vi "Stop Server.vi"(8 "error in (no error)":errorcluster, 11 "OOP Server in":refnum<class "Template Server.lvclass">) -> (0 "error out":errorcluster, 3 "OOP Server out":refnum<class "Template Server.lvclass">)   [LabVIEW 2019, in "Template Server.lvlib" / "Template Server.lvclass"]
uses:
  Template Server.lvclass
  Template Server.lvclass/Template Server.ctl
  gRPC interface/gprc-lvsupport.lvlib
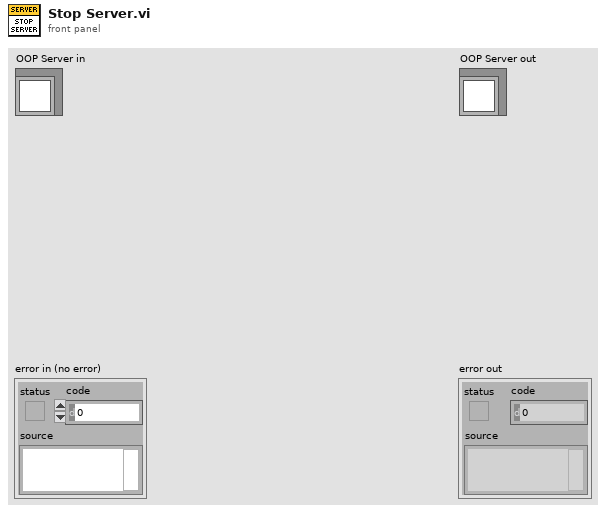
[diagram p1: front panel]
types:
  T1 = typedef "gprc-lvsupport.lvlib/grpcId.ctl" = u64
  T2 = typedef "Template Server.lvlib/Template Server.lvclass/Server gRPC UEs.ctl" = cluster{"Template gRPCId UE":T3}
  T3 = typedef "gprc-lvsupport.lvlib/gRPCId Cluster UE.ctl" = refnum<user-event>
  T4 = typedef "Template Server.lvlib/Template Server.lvclass/Server Internal UEs.ctl" = cluster{"Template Internal UE":refnum<user-event>}
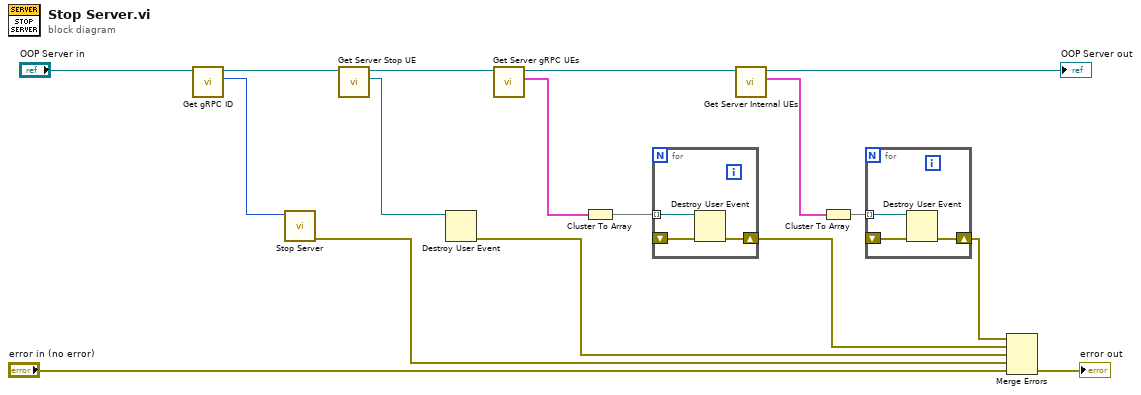
[diagram p0: block diagram]
diagram:
  n1 = call "Get gRPC ID.vi"("OOP Server in"="OOP Server in") -> ("gRPC ID"=w15:T1, "OOP Server out"=w14:refnum<class "Template Server.lvclass">)  [unwired: 9 in]
  n2 = call "Stop Server.vi"("Server Id"=w15) -> ("error out"=w1:errorcluster)  [unwired: 10 in]
  n3 = call "Get Server Stop UE.vi"("OOP Server in"=w14) -> ("Server Stop UE"=w13:refnum<user-event>, "OOP Server out"=w12:refnum<class "Template Server.lvclass">)  [unwired: 9 in]
  n4 = Destroy User Event(user event=w13) -> (error out=w2:errorcluster)  [unwired: 1 in]
  n5 = call "Get Server gRPC UEs.vi"("OOP Server in"=w12) -> ("Server gRPC UEs"=w10:T2, "OOP Server out"=w11:refnum<class "Template Server.lvclass">)  [unwired: 9 in]
  n6 = Cluster To Array(cluster=w10) -> (array=w9:T3[])
  n7 = for {
    tunnel: w9 -> [w20] mode=indexing
    shift-right: [w18] -> w3
    shift-left: _ -> [w19]
    n8 = Destroy User Event(user event=w20, error in=w19) -> (error out=w18:errorcluster)
  }
  n9 = call "Get Server Internal UEs.vi"("OOP Server in"=w11) -> ("Server Internal UEs"=w8:T4, "OOP Server out"=→"OOP Server out":refnum<class "Template Server.lvclass">)  [unwired: 9 in]
  n10 = Cluster To Array(cluster=w8) -> (array=w7:refnum<user-event>[])
  n11 = for {
    tunnel: w7 -> [w23] mode=indexing
    shift-right: [w21] -> w4
    shift-left: _ -> [w22]
    n12 = Destroy User Event(user event=w23, error in=w22) -> (error out=w21:errorcluster)
  }
  n13 = Merge Errors(w4, w3, w2, w1, "error in (no error)") -> (→"error out":errorcluster)
